vi "test sequencer.vi"(8 "error in (no error)":errorcluster, 11 "this module name":string) -> (0 "error out":errorcluster)   [LabVIEW 2019]
uses:
  common/common data types/common_event_data.ctl
panel:
  out "global stop?":bool
  in  "stop this module":bool
  out "targetted":bool
  out "msg target":string
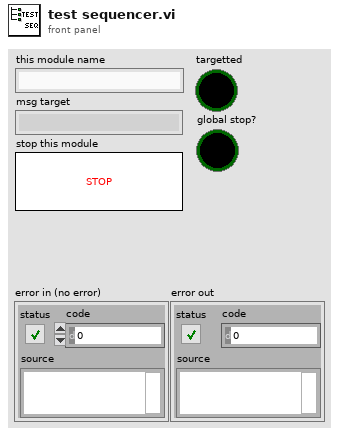
[diagram p1: front panel]
types:
  T1 = typedef "common_event_data.ctl" = cluster{"sender":string, "target":string, "msg":string, "data":variant}
  T2 = cluster{"this module name":string, "example data":bool, "test seq path":path, "test seq parsed":string[][]}
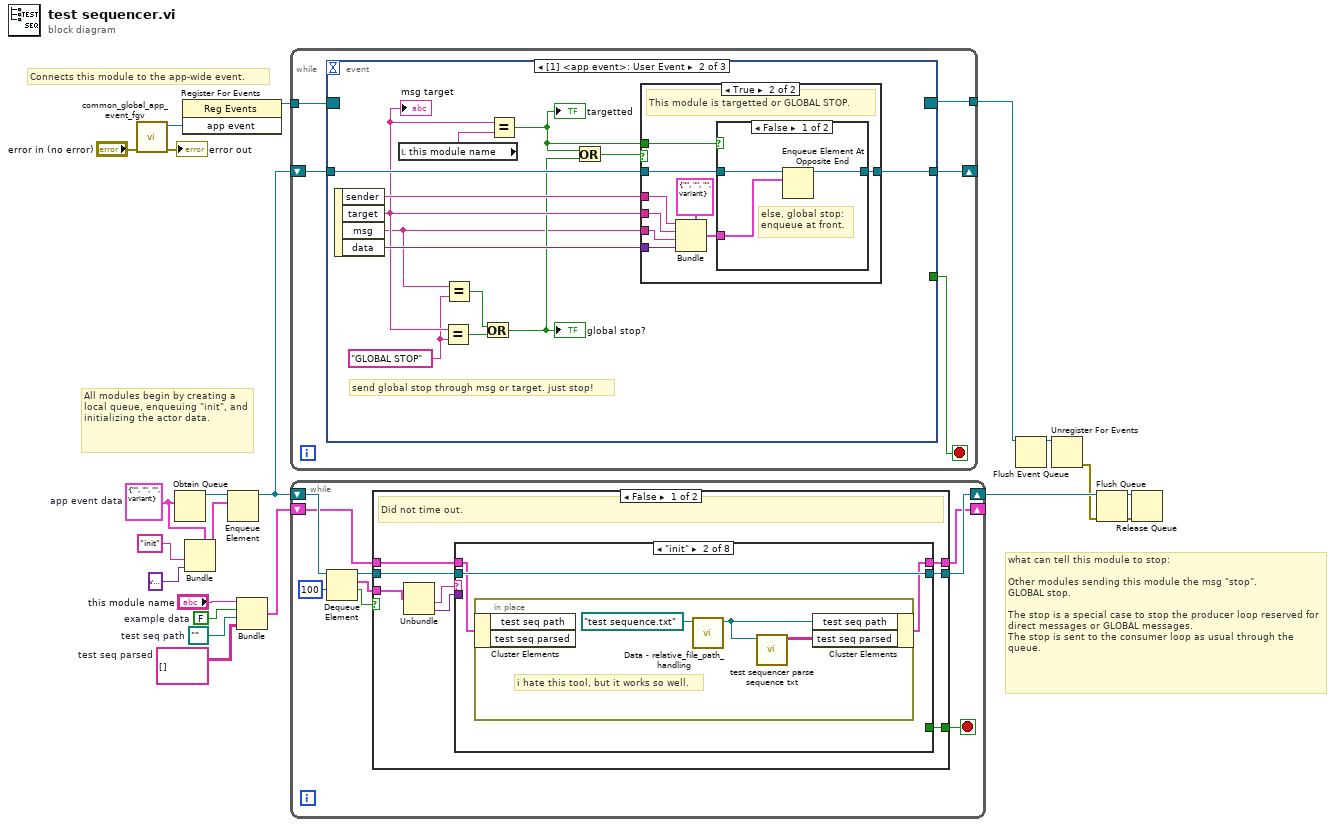
[diagram p0: block diagram]
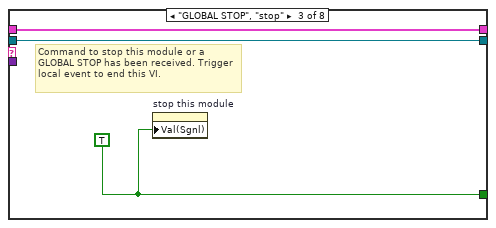
[diagram p3: hidden frame]
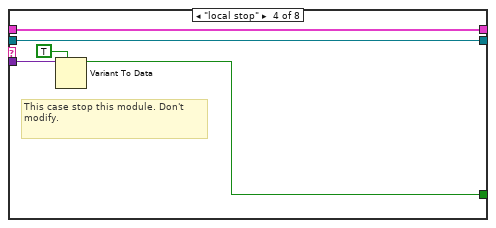
[diagram p4: hidden frame]
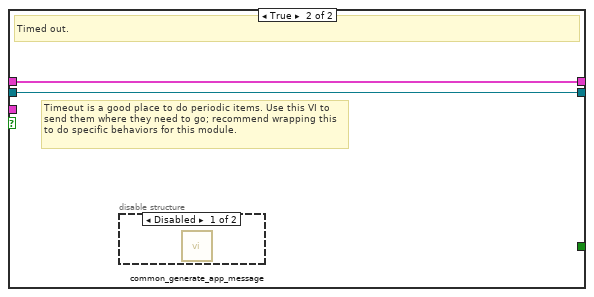
[diagram p9: hidden frame]
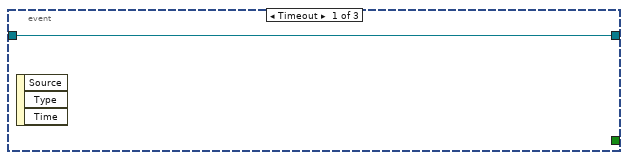
[diagram p11: hidden frame]
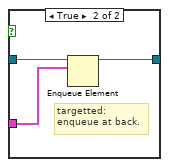
[diagram p13: hidden frame]
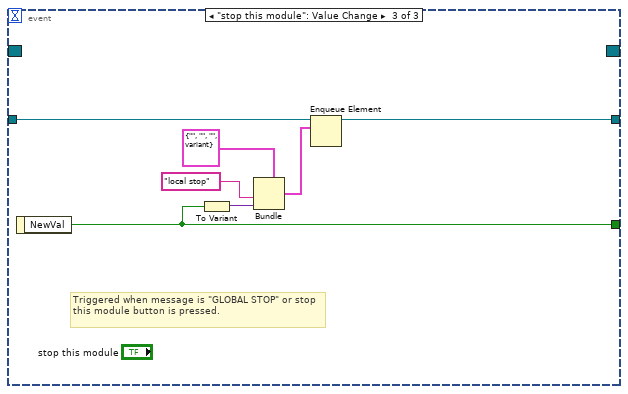
[diagram p14: hidden frame]
diagram:
  w2 = string[][] []  # test seq parsed
  w3 = path ""  # test seq path
  w7 = FALSE  # example data
  w10 = T1 {"sender"="", "target"="", "msg"="", "data"=variant}  # app event data
  # "All modules begin by creating a local queue, enqueuing \"init\", and initializing the actor data."
  # "what can tell this module to stop:\n\nOther modules sending this module the msg \"stop\".\nGLOBAL stop.\n\nThe stop is a special case to stop the producer loop reserved for direct messages or GLOBAL messages.\nThe stop is sent to the consumer loop as usual through the queue."
  # "Connects this module to the app-wide event."
  n1 = call "common_global_app_event_fgv.vi"("error in (no error)"="error in (no error)") -> ("error out"=→"error out":errorcluster, "app event"=w15:refnum<user-event>)  [unwired: 9 in]
  n2 = Obtain Queue(element data type=w10) -> (queue out=w21:refnum<queue>)  [unwired: 4 in, 2 out]
  n3 = register-events(w15) -> (reference out=w16:refnum<event-registration>)  [unwired: 2 in, 1 out]
  n4 = Bundle(cluster=w10, "msg"="init", "data"=variant) -> (w20:T1)  [unwired: 2 in]
  n5 = Enqueue Element(queue=w21, element=w20) -> (queue out=w19:refnum<queue>)  [unwired: 2 in, 2 out]
  n6 = Bundle("this module name"="this module name", "example data"=w7, "test seq path"=w3, "test seq parsed"=w2) -> (w6:T2)  [unwired: 1 in]
  n7 = while {
    tunnel: w16 -> [w26]
    shift-right: [w24] -> _
    shift-left: w19 -> [w25]
    tunnel: [w23] -> w5
    stop <- w22 stop-if-true
    n8 = event shown="[1] <app event>: User Event" {
      selector: w26 -> [_ _ _]
      dyn-events: [_ _ _] -> w23
      timeout: _ -> [_ _ _]
      tunnel: w25 -> [w27 w39 w61]
      tunnel: [w27 w38 w62] -> w24
      tunnel: [_ _ w57] -> w22
      event Timeout {
        n9 = event-data() -> ()  [unwired: 1 in, 3 out]
      }
      event User Event {
        w31 = "GLOBAL STOP"
        # "send global stop through msg or target. just stop!"
        n10 = event-data() -> ("sender"=w37:string, "target"=w36:string, "msg"=w30:string, "data"=w40:variant)  [unwired: 1 in]
        "msg target" <- w36
        n11 = local read "this module name"() -> (w28:string)
        n12 = Equal?(x=w36, y=w31) -> (x = y?=w33:bool)
        n13 = Equal?(x=w30, y=w31) -> (x = y?=w29:bool)
        n14 = Or(x=w29, y=w33) -> (x .or. y?=w32:bool)
        "global stop?" <- w32
        n15 = Equal?(x=w36, y=w28) -> (x = y?=w34:bool)
        "targetted" <- w34
        n16 = Or(x=w34, y=w32) -> (x .or. y?=w35:bool)
        n17 = case shown="True" w35 {
          tunnel: w30 -> [_ w46]
          tunnel: w40 -> [_ w47]
          tunnel: w39 -> [w41 w50]
          tunnel: [w41 w49] -> w38
          tunnel: w36 -> [_ w45]
          tunnel: w37 -> [_ w44]
          tunnel: w34 -> [_ w42]
          frame False {
          }
          frame True {
            # "This module is targetted or GLOBAL STOP."
            n18 = Bundle(cluster=T1 {"sender"="", "target"="", "msg"="", "data"=variant}, "sender"=w44, "target"=w45, "msg"=w46, "data"=w47) -> (w43:T1)
            n19 = case shown="False" w42 {
              tunnel: w50 -> [w53 w56]
              tunnel: [w52 w55] -> w49
              tunnel: w43 -> [w51 w54]
              frame False {
                # "else, global stop: \nenqueue at front."
                n20 = Enqueue Element At Opposite End(queue=w53, element=w51) -> (queue out=w52:refnum<queue>)  [unwired: 2 in, 2 out]
              }
              frame True {
                # "targetted:\nenqueue at back."
                n21 = Enqueue Element(queue=w56, element=w54) -> (queue out=w55:refnum<queue>)  [unwired: 2 in, 2 out]
              }
            }
          }
        }
      }
      event "stop this module": Value Change {
        # "Triggered when message is \"GLOBAL STOP\" or stop this module button is pressed."
        n22 = event-data() -> ("NewVal"=w57:bool)  [unwired: 1 in]
        n23 = To Variant(anything=w57) -> (Variant=w58:variant)
        n24 = Bundle(cluster=T1 {"sender"="", "target"="", "msg"="", "data"=variant}, "msg"="local stop", "data"=w58) -> (w63:T1)  [unwired: 2 in]
        n25 = Enqueue Element(queue=w61, element=w63) -> (queue out=w62:refnum<queue>)  [unwired: 2 in, 2 out]
      }
    }
  }
  n26 = while {
    shift-right: [w69] -> w17
    shift-left: w19 -> [w72]
    shift-right: [w64] -> _
    shift-left: w6 -> [w65]
    stop <- w68 stop-if-true
    n27 = Dequeue Element(queue=w72, timeout in ms (-1)=100) -> (queue out=w70:refnum<queue>, element=w71:T1, timed out?=w67:bool)  [unwired: 1 in, 1 out]
    n28 = case shown="False" w67 {
      tunnel: w71 -> [w80 _]
      tunnel: w70 -> [w79 w106]
      tunnel: [w78 w106] -> w69
      tunnel: [w77 _] -> w68
      tunnel: w65 -> [w74 w105]
      tunnel: [w73 w105] -> w64
      frame False {
        # "Did not time out."
        n29 = Unbundle(w80) -> ("msg"=w75:string, "data"=w76:variant)  [unwired: 2 out]
        n30 = case shown="\"init\"" w75 {
          tunnel: w79 -> [w82 w85 w91 w96 w98 w100 w102 w104]
          tunnel: [w82 w85 w91 w96 w98 w100 w102 w104] -> w78
          tunnel: w76 -> [_ _ _ w94 _ _ _ _]
          tunnel: [_ _ w90 w93 _ _ _ _] -> w77
          tunnel: w74 -> [w81 w84 w89 w92 w97 w99 w101 w103]
          tunnel: [w81 w83 w89 w92 w97 w99 w101 w103] -> w73
          frame "---Core VIs---" {
            # "In general, do not modify these cases. I've added #exception where custom behavior is encouraged/expected."
          }
          frame "init" {
            n31 = in-place {
              # "i hate this tool, but it works so well."
              n32 = in-place-cluster #1(w84) -> ()  [unwired: 2 out]
              n33 = call "Data - relative_file_path_handling.vi"("path in"=path "test sequence.txt") -> ("path out"=w86:path)  [unwired: 9 in, 1 out]
              n34 = call "test sequencer parse sequence txt.vi"("sequence txt path"=w86) -> ("steps"=w87:string[][])  [unwired: 9 in, 1 out]
              n35 = in-place-cluster #1("test seq path"=w86, "test seq parsed"=w87) -> (w83:T2)
            }
          }
          frame "GLOBAL STOP", "stop" {
            w90 = TRUE
            # "Command to stop this module or a GLOBAL STOP has been received. Trigger local event to end this VI."
            n36 = property on="stop this module" class="Bool (strict)"("Val(Sgnl)"=w90) -> ()  [unwired: 2 in, 2 out]
          }
          frame "local stop" {
            # "This case stop this module. Don't modify."
            n37 = Variant To Data(type=TRUE, Variant=w94) -> (data=w93:bool)  [unwired: 1 in, 1 out]
          }
          frame "---Test Steps---" {
            # "In this section, you would put behaviors specific to your module."
          }
          frame Default {
            # "unsupported message."
          }
          frame "action1 " {
            # "Have this module do something here!"
          }
          frame "action2" {
            # "Have this module do something here, too!"
          }
        }
      }
      frame True {
        # "Timeout is a good place to do periodic items. Use this VI to send them where they need to go; recommend wrapping this to do specific behaviors for this module."
        # "Timed out."
        n38 = disable-structure shown="Disabled" {
          frame Disabled {
            n39 = call "common_generate_app_message.vi"() -> ()  [unwired: 11 in, 1 out]
          }
          frame Enabled {
          }
        }
      }
    }
  }
  n40 = Flush Event Queue(0:w5) -> (8:w4:refnum<event-registration>)  [unwired: 5 in, 2 out]
  n41 = Unregister For Events(event registration refnum=w4) -> (error out=w12:errorcluster)  [unwired: 1 in]
  n42 = Flush Queue(queue=w17, error in (no error)=w12) -> (queue out=w18:refnum<queue>, error out=w11:errorcluster)  [unwired: 1 out]
  n43 = Release Queue(queue=w18, error in (no error)=w11) -> ()  [unwired: 1 in, 3 out]
